vi "SRV_Read_Comm_Response after Reboot.vi"(8 "error in (no error)":errorcluster, 11 "SRV In":refnum<k5>) -> (0 "error out":errorcluster, 2 "Data out":string, 3 "SRV Out":refnum<k5>)   [LabVIEW 2009]
uses:
  TCP_Communication/SRV_TCP Settings.ctl
  TCP_Communication/SRV_Package Methods.ctl
panel:
  out "Data 2":string
  out "Data 1":string
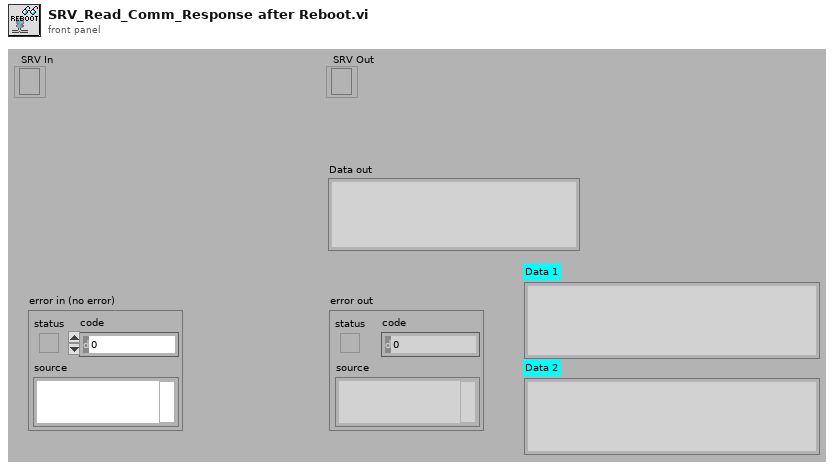
[diagram p1: front panel]
types:
  T1 = typedef "SRV_TCP Settings.ctl" = cluster{"Method":T2, "bytes to read":i32, "timeout ms (1000)":i32}
  T2 = typedef "SRV_Package Methods.ctl" = enum16{"General", "Standard", "CRLF", "Image", "HTML"}
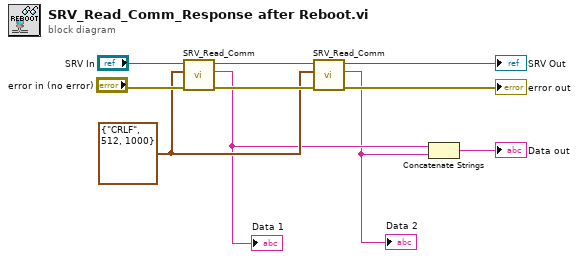
[diagram p0: block diagram]
diagram:
  w5 = T1 {"Method"=enum."CRLF", "bytes to read"=512, "timeout ms (1000)"=1000} ("TCP Settings")
  n1 = call "SRV_Read_Comm.vi"("error in (no error)"="error in (no error)", "TCP Settings"=w5, "SRV In"="SRV In") -> ("error out"=w7:errorcluster, "Data out"=w3:string, "SRV Out"=w9:refnum<k5>)  [unwired: 6 in]
  "Data 1" <- w3
  n2 = call "SRV_Read_Comm.vi"("error in (no error)"=w7, "TCP Settings"=w5, "SRV In"=w9) -> ("error out"=→"error out":errorcluster, "Data out"=w1:string, "SRV Out"=→"SRV Out":refnum<k5>)  [unwired: 6 in]
  "Data 2" <- w1
  n3 = Concatenate Strings(w3, w1) -> (→"Data out":string)
